vi "Randomize_trials.vi"(10 "Repeats":u32, 11 "Protocol cluster":T1) -> (3 "Trials":string[](array[string]))   [LabVIEW 2016]
uses:
  <vilib>/Analysis/1siggen.llb/Riffle Array (I32).vi
  <vilib>/Analysis/NI_AALBase.lvlib
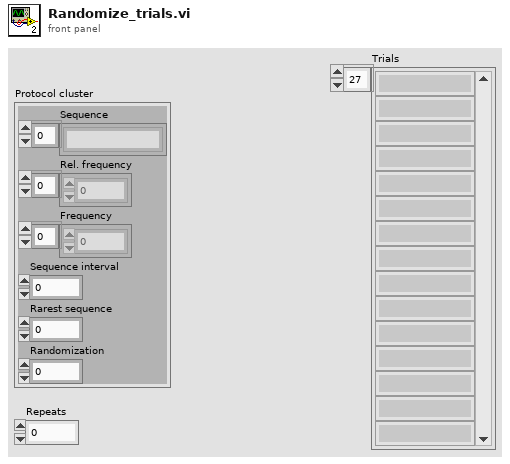
[diagram p1: front panel]
types:
  T1 = cluster{"Sequence":string[], "Rel. frequency":u32[], "Frequency":dbl[], "Sequence interval":dbl, "Rarest sequence ":dbl, "Randomization":u16}
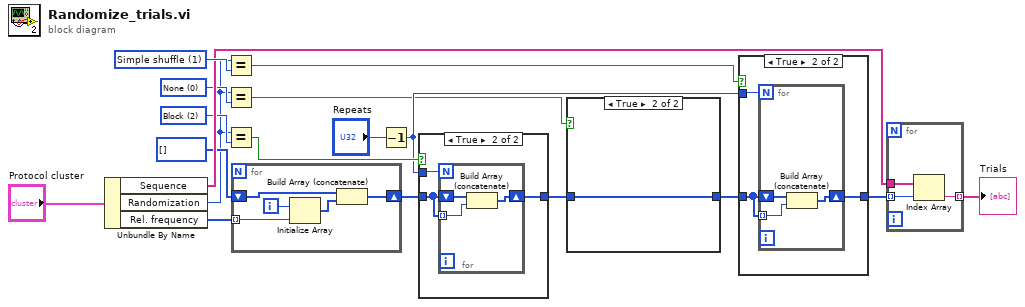
[diagram p0: block diagram]
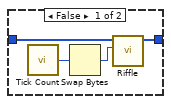
[diagram p2: hidden frame]
diagram:
  w3 = u16 0 items=["None", "Simple shuffle", "Block"] ("Randomization")
  w14 = u16 1 items=["None", "Simple shuffle", "Block"] ("Randomization")
  w9 = u16 2 items=["None", "Simple shuffle", "Block"] ("Randomization")
  n1 = Unbundle By Name("Protocol cluster") -> ("Sequence"=w13:string[], "Randomization"=w2:u16, "Rel. frequency"=w7:u32[])
  n2 = Equal?(x=w2, y=w14) -> (x = y?=w15:bool)
  n3 = Equal?(x=w2, y=w3) -> (x = y?=w1:bool)
  n4 = Equal?(x=w2, y=w9) -> (x = y?=w10:bool)
  n5 = for {
    tunnel: w7 -> [w21] mode=indexing
    shift-right: [w22] -> w11
    shift-left: u32[] [] ("Rel. requency") -> [w23]
    i -> [w20]
    n6 = Initialize Array(w20, w21) -> (w19:i32[])
    n7 = Build Array (concatenate)(w23, w19) -> (w22:u32[])
  }
  n8 = Decrement(x="Repeats") -> (x-1=w4:u32)
  n9 = case shown="True" w10 {
    tunnel: w11 -> [w24 w26]
    tunnel: w4 -> [_ w27]
    tunnel: [w24 w25] -> w12
    frame False {
    }
    frame True {
      n10 = for {
        N: w27 -> [_]
        shift-right: [w28] -> w25
        shift-left: w26 -> [w30]
        tunnel: w26 -> [w29] mode=indexing
        n11 = Build Array (concatenate)(w30, w29) -> (w28:u32[])
      }
    }
  }
  n12 = case shown="True" w1 {
    tunnel: [w34 w35] -> w16
    tunnel: w12 -> [w33 w35]
    frame False {
      n13 = call "Tick Count"() -> ("Tick Count(Ticks)"=w31:u32)
      n14 = Swap Bytes(anything=w31) -> (byte swapped=w32:u32)
      n15 = call-poly <vilib>:"Riffle.vi"("seed"=w32, "X"=w33) -> ("Riffled {X}"=w34:i32[])  [unwired: 7 in, 2 out]
    }
    frame True {
    }
  }
  n16 = case shown="True" w15 {
    tunnel: w16 -> [w36 w38]
    tunnel: w4 -> [_ w39]
    tunnel: [w36 w37] -> w18
    frame False {
    }
    frame True {
      n17 = for {
        N: w39 -> [_]
        shift-right: [w40] -> w37
        shift-left: w38 -> [w42]
        tunnel: w38 -> [w41] mode=indexing
        n18 = Build Array (concatenate)(w42, w41) -> (w40:u32[])
      }
    }
  }
  n19 = for {
    tunnel: w18 -> [w44] mode=indexing
    tunnel: w13 -> [w45]
    tunnel: [w43] -> w5 mode=indexing
    n20 = Index Array(array=w45, index=w44) -> (element=w43:string)
  }
  "Trials" <- w5
